vi "Singulator Teleop.vi"(11 "Setpoint":bool) -> ()   [LabVIEW 2019]
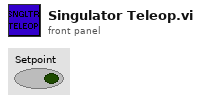
[diagram p1: front panel]
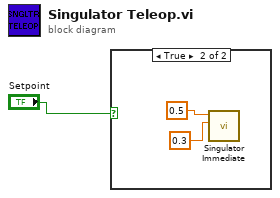
[diagram p0: block diagram]
diagram:
  n1 = case shown="True" "Setpoint" {
    frame False {
    }
    frame True {
      n2 = call "Singulator Immediate.vi"("Right Setpoint"=0.3, "Left Setpoint"=0.5) -> ()  [unwired: 9 in, 1 out]
    }
  }
